vi "LM formula string function.vi"(3 "output control":T1, 4 "function parameters":variant, 5 "X":dbl[](array[numeric]), 6 "a":dbl[](array[numeric])) -> (0 "error out":errorcluster, 1 "f'(X)":dbl[][](array[numeric]), 2 "f(X)":dbl[](array[numeric]))   [LabVIEW 2017, in "NI_Gmath.lvlib"]
uses:
  <vilib>/gmath/NI_Gmath.lvlib
  <vilib>/gmath/NumericalOptimization/LM_output select.ctl
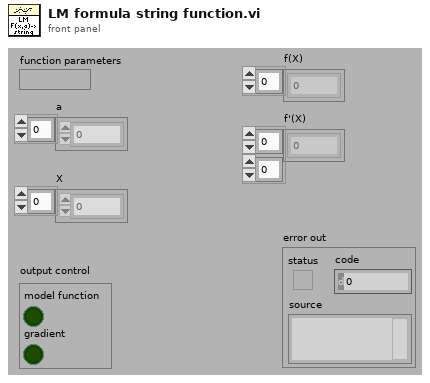
[diagram p1: front panel]
types:
  T1 = typedef "NI_Gmath.lvlib/LM_output select.ctl" = cluster{"model function":bool, "gradient":bool}
  T2 = cluster{"model":string, "Parameters":string[], "x":string}
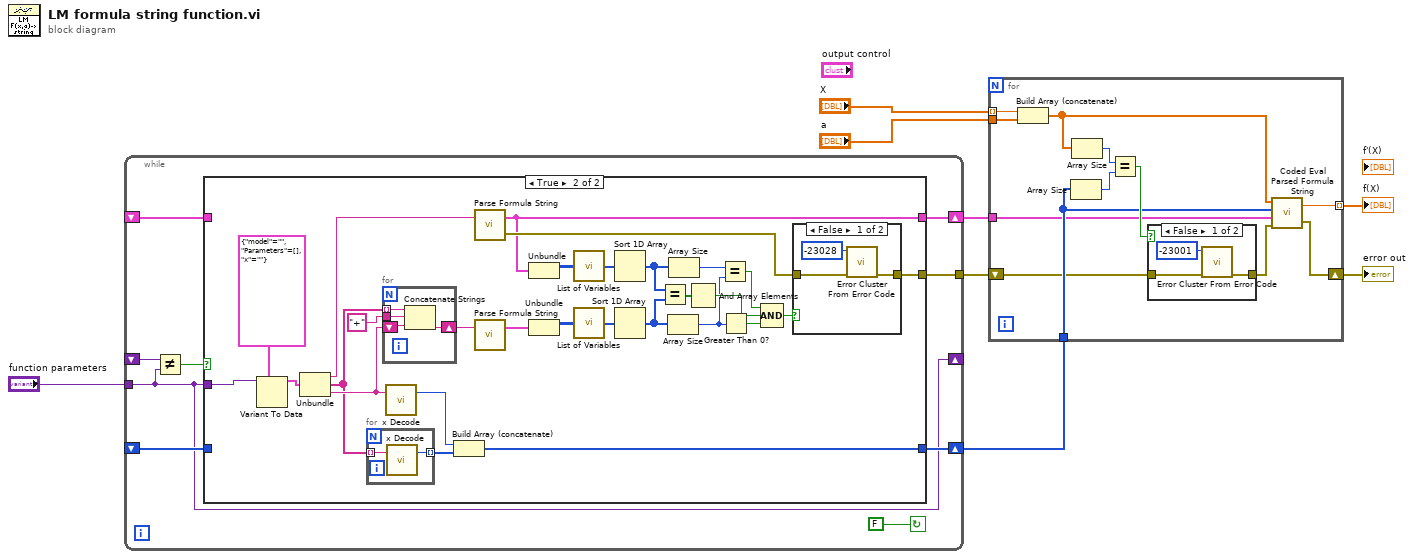
[diagram p0: block diagram]
diagram:
  n1 = while {
    shift-right: [w14] -> w2
    shift-left: _ -> [w13]
    shift-right: [w16] -> w3
    shift-left: _ -> [w15]
    tunnel: [w12] -> w1
    tunnel: "function parameters" -> [w10]
    shift-right: [w10] -> _
    shift-left: _ -> [w9]
    stop <- FALSE continue-if-true
    n2 = Not Equal?(x=w9, y=w10) -> (x != y?=w11:bool)
    n3 = case shown="True" w11 {
      tunnel: [w19 w31] -> w16
      tunnel: w15 -> [w19 _]
      tunnel: [w18 w30] -> w14
      tunnel: w13 -> [w18 _]
      tunnel: [_ w29] -> w12
      tunnel: w10 -> [_ w26]
      frame False {
      }
      frame True {
        n4 = Variant To Data(type=T2 {"model"="", "Parameters"=[], "x"=""} ("model description"), Variant=w26) -> (data=w27:T2)  [unwired: 1 in, 1 out]
        n5 = Unbundle(w27) -> ("model"=w46:string, "Parameters"=w44:string[], "x"=w45:string)
        n6 = for {
          tunnel: w44 -> [w57] mode=indexing
          tunnel: [w56] -> w38 mode=indexing
          n7 = call <vilib>:"x Decode.vi"("x string"=w57) -> ("number"=w56:i32)  [unwired: 1 in, 1 out]
        }
        n8 = for {
          shift-right: [w52] -> w37
          shift-left: w45 -> [w53]
          tunnel: w44 -> [w55] mode=indexing
          tunnel: "+" -> [w54]
          n9 = Concatenate Strings(w55, w54, w53) -> (w52:string)
        }
        n10 = call <vilib>:"x Decode.vi"("x string"=w45) -> ("number"=w47:i32)  [unwired: 1 in, 1 out]
        n11 = Build Array (concatenate)(w47, w38) -> (w31:i32[])
        n12 = call <vilib>:"Parse Formula String.vi"("formula"=w46) -> ("error out"=w32:errorcluster, "Parsed Formula"=w30:cluster{"Table":i32[][], "Y Values":dbl[]})  [unwired: 1 in]
        n13 = call <vilib>:"Parse Formula String.vi"("formula"=w37) -> ("Parsed Formula"=w36:cluster{"Table":i32[][], "Y Values":dbl[]})  [unwired: 1 in, 1 out]
        n14 = Unbundle(w30) -> ("Table"=w35:i32[][])  [unwired: 1 out]
        n15 = Unbundle(w36) -> ("Table"=w34:i32[][])  [unwired: 1 out]
        n16 = call <vilib>:"List of Variables.vi"("Table"=w35) -> ("List of variables"=w42:i32[])
        n17 = call <vilib>:"List of Variables.vi"("Table"=w34) -> ("List of variables"=w43:i32[])
        n18 = Sort 1D Array(array=w42) -> (sorted array=w22:i32[])
        n19 = Sort 1D Array(array=w43) -> (sorted array=w23:i32[])
        n20 = Equal?(x=w22, y=w23) -> (x = y?=w41:bool[])
        n21 = Array Size(array=w23) -> (size(s)=w20:i32)
        n22 = Array Size(array=w22) -> (size(s)=w21:i32)
        n23 = And Array Elements(Boolean array=w41) -> (logical AND=w40:bool)
        n24 = Equal?(x=w21, y=w20) -> (x = y?=w25:bool)
        n25 = Greater Than 0?(x=w20) -> (x > 0?=w24:bool)
        n26 = Compound Arithmetic op=AND(w25, w40, w24) -> (w33:bool)
        n27 = case shown="False" w33 {
          tunnel: w32 -> [w49 w51]
          tunnel: [w48 w51] -> w29
          frame False {
            n28 = call <vilib>:"Error Cluster From Error Code.vi"("error in (no error)"=w49, "error code (0)"=-23028) -> ("error out"=w48:errorcluster)  [unwired: 7 in]
          }
          frame True {
          }
        }
      }
    }
  }
  n29 = for {
    tunnel: [w67] -> w8 mode=indexing
    tunnel: "a" -> [w63]
    tunnel: "X" -> [w62] mode=indexing
    tunnel: w3 -> [w60]
    tunnel: w2 -> [w59]
    shift-right: [w64] -> w7
    shift-left: w1 -> [w58]
    n30 = Build Array (concatenate)(w62, w63) -> (w61:dbl[])
    n31 = Array Size(array=w60) -> (size(s)=w68:i32)
    n32 = Array Size(array=w61) -> (size(s)=w69:i32)
    n33 = Equal?(x=w69, y=w68) -> (x = y?=w66:bool)
    n34 = case shown="False" w66 {
      tunnel: w58 -> [w71 w73]
      tunnel: [w70 w73] -> w65
      frame False {
        n35 = call <vilib>:"Error Cluster From Error Code.vi"("error in (no error)"=w71, "error code (0)"=-23001) -> ("error out"=w70:errorcluster)  [unwired: 7 in]
      }
      frame True {
      }
    }
    n36 = call <vilib>:"Coded Eval Parsed Formula String.vi"("error in (no error)"=w65, "Parsed Formula"=w59, "Variables"=w60, "X Values"=w61) -> ("error out"=w64:errorcluster, "y value"=w67:dbl)
  }
  "f(X)" <- w8
  "error out" <- w7
